vi "mMc - global.vi"() -> ()   [LabVIEW 2011]
panel:
  out "done":bool
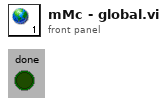
[diagram p1: front panel]
diagram:
